vi "Error Add Info.vi"(8 "error in":errorcluster, 9 "Info":string) -> (0 "error out":errorcluster)   [LabVIEW 2020, in "g-sugar.lvlib"]
doc: "Inserts an <b>info</b> string into the <b>error in</b> source message. If there is no error / warning, no modifications are made to the <b>error out</b>."
uses:
  g-sugar.lvlib
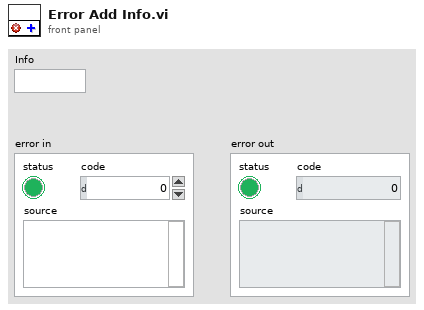
[diagram p1: front panel]
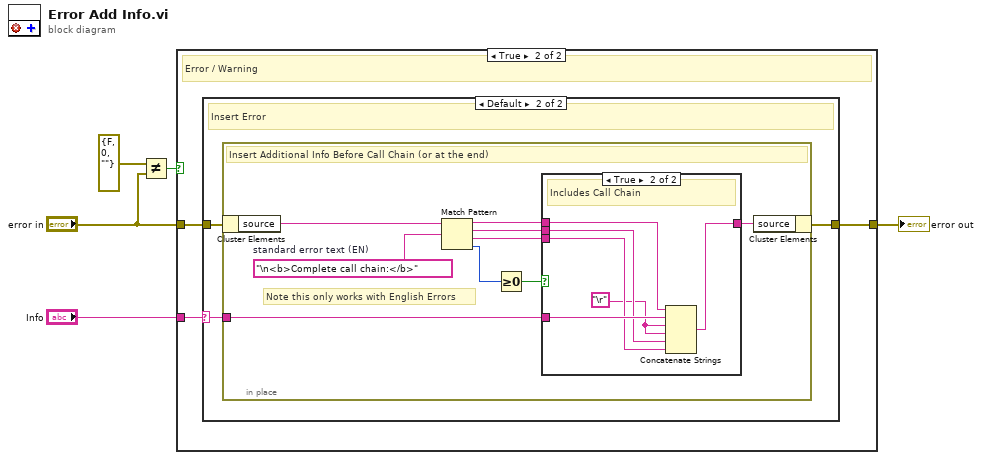
[diagram p0: block diagram]
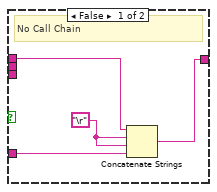
[diagram p4: hidden frame]
diagram:
  n1 = Not Equal?(x=errorcluster {"status"=FALSE, "code"=0, "source"=""}, y="error in") -> (x != y?=w1:bool)
  n2 = case shown="True" w1 {
    tunnel: [w6 w8] -> w5
    tunnel: "Info" -> [_ w7]
    tunnel: "error in" -> [w6 w9]
    frame False {
      # "NOT Error or Warning"
    }
    frame True {
      # "Error / Warning"
      n3 = case shown="Default" w7 {
        selector: w7 -> [_ w11]
        tunnel: w9 -> [w10 w13]
        tunnel: [w10 w12] -> w8
        frame "" {
          # "Empty String, Don't Modify the Error"
        }
        frame Default {
          # "Insert Error"
          n4 = in-place {
            in-place-border: w11 -> [w21]
            w19 = "\n<b>Complete call chain:</b>"  # standard error text (EN)
            # "Note this only works with English Errors"
            # "Insert Additional Info Before Call Chain (or at the end)"
            n5 = in-place-cluster #1(w13) -> ("source"=w20:string)
            n6 = Match Pattern(string=w20, regular expression=w19) -> (before substring=w16:string, match substring=w17:string, after substring=w18:string, offset past match=w15:i32)  [unwired: 1 in]
            n7 = Greater Or Equal To 0?(x=w15) -> (x >= 0?=w14:bool)
            n8 = case shown="True" w14 {
              tunnel: [w25 w32] -> w22
              tunnel: w21 -> [w23 w31]
              tunnel: w18 -> [_ w30]
              tunnel: w17 -> [_ w29]
              tunnel: w16 -> [w26 w28]
              frame False {
                w24 = "\r"
                # "No Call Chain"
                n9 = Concatenate Strings(w26, w24, w24, w23) -> (w25:string)
              }
              frame True {
                w27 = "\r"
                # "Includes Call Chain"
                n10 = Concatenate Strings(w28, w31, w27, w27, w29, w30) -> (w32:string)
              }
            }
            n11 = in-place-cluster #1("source"=w22) -> (w12:errorcluster)
          }
        }
      }
    }
  }
  "error out" <- w5
